vi "Write Roles.vi"(8 "error in (no error)":errorcluster, 10 "Roles":T1, 11 "DirectKickPlay in":refnum<class "DirectKickPlay.lvclass">) -> (0 "error out":errorcluster, 3 "DirectKickPlay out":refnum<class "DirectKickPlay.lvclass">)   [LabVIEW 2018, in "DirectKickPlay.lvclass"]
uses:
  DirectKickPlay.lvclass
  FollowAttackerRole_class/FollowAttackerRole.lvclass
  ShootRole_class/ShootRole.lvclass
  DirectKickPlay.lvclass/DirectKickPlay.ctl
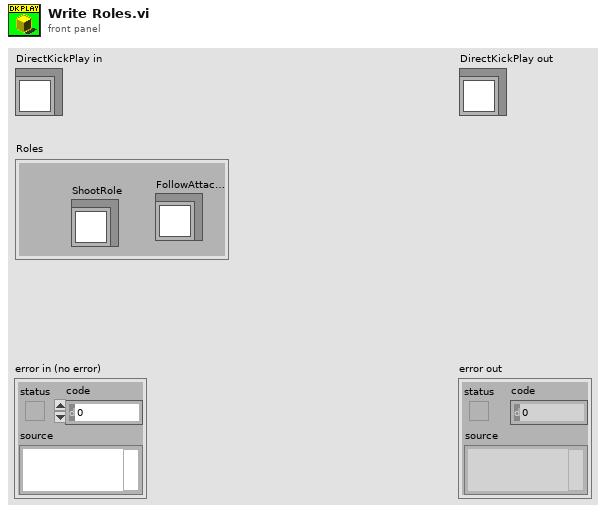
[diagram p1: front panel]
types:
  T1 = cluster{"FollowAttackerRole":refnum<class "FollowAttackerRole.lvclass">, "ShootRole":refnum<class "ShootRole.lvclass">}
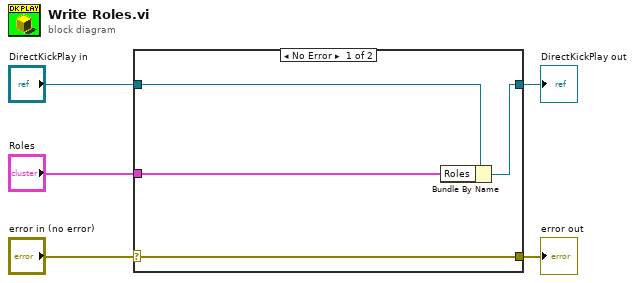
[diagram p0: block diagram]
diagram:
  n1 = case shown="No Error" "error in (no error)" {
    selector: "error in (no error)" -> [w9 w10]
    tunnel: [w9 w10] -> w4
    tunnel: [w7 w11] -> w2
    tunnel: "DirectKickPlay in" -> [w8 w11]
    tunnel: "Roles" -> [w6 _]
    frame No Error {
      n2 = Bundle By Name(cluster=w8, "Roles"=w6) -> (w7:refnum<class "DirectKickPlay.lvclass">)
    }
    frame Error {
    }
  }
  "error out" <- w4
  "DirectKickPlay out" <- w2
